vi "png path to tdms image path.vi"(11 "png path":path) -> (3 "tdms image path":path)   [LabVIEW 2018]
panel:
  out "ScanFolderName":string
  out "Dev name":string
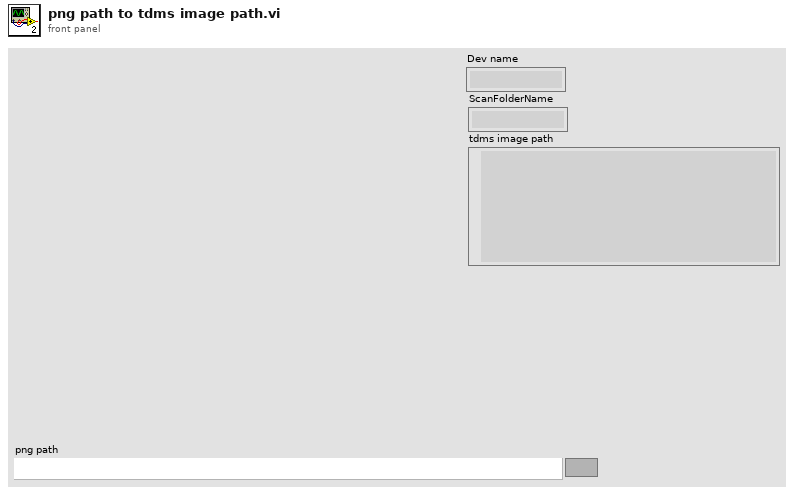
[diagram p1: front panel]
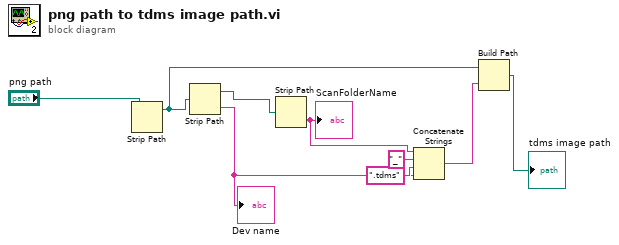
[diagram p0: block diagram]
diagram:
  n1 = Strip Path(path="png path") -> (stripped path=w1:path)  [unwired: 1 out]
  n2 = Strip Path(path=w1) -> (stripped path=w9:path, name=w6:string)
  "Dev name" <- w6
  n3 = Strip Path(path=w9) -> (name=w7:string)  [unwired: 1 out]
  "ScanFolderName" <- w7
  n4 = Concatenate Strings(w7, "_" ("string"), w6, ".tdms" ("string")) -> (w3:string)
  n5 = Build Path(base path=w1, name or relative path=w3) -> (appended path=→"tdms image path":path)
